vi "DSF.Engine.Plugin.Return Transfer Group.vi"(8 "error in (no error)":errorcluster, 10 "Transfer Group":refnum<class "DSF.Engine.Transfer Group.lvclass">, 11 "Plugin in":refnum<class "DSF.Engine.Plugin.lvclass">) -> (0 "error out":errorcluster, 3 "Plugin out":refnum<class "DSF.Engine.Plugin.lvclass">)   [LabVIEW 2017, in "DSF.Engine.lvlib" / "DSF.Engine.Plugin.lvclass"]
uses:
  DSF.Engine.Plugin.lvclass
  Transfer/DSF.Engine.Transfer Group.lvclass
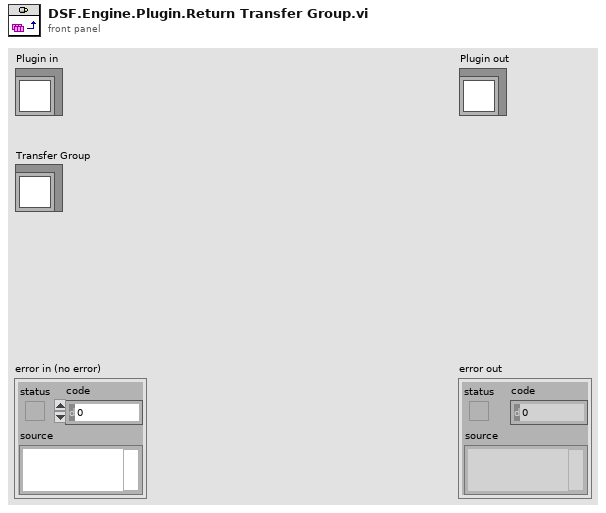
[diagram p1: front panel]
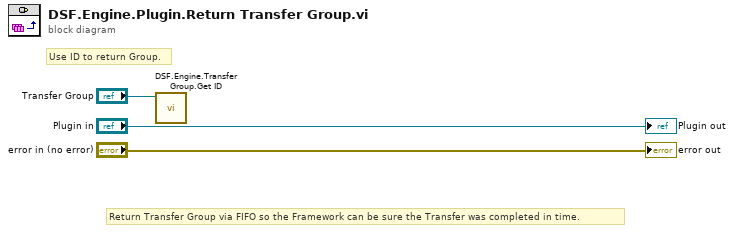
[diagram p0: block diagram]
diagram:
  # "Return Transfer Group via FIFO so the Framework can be sure the Transfer was completed in time."
  # "Use ID to return Group."
  n1 = call "DSF.Engine.Transfer Group.Get ID.vi"("Transfer Group in"="Transfer Group") -> ()  [unwired: 9 in, 2 out]
  "error out" <- "error in (no error)"
  "Plugin out" <- "Plugin in"
